vi "Example Callback - UVI Callback.vi"(4 "UVI":refnum<user-event>, 5 "Event Data":cluster{"sender":refnum<k24>, "uvi":i32}, 6 "Control Ref":refnum<k24>, 7 "Event Common Data":T1) -> ()   [LabVIEW 2010]
uses:
  C:/tf/play/labview/Tinkerforge.dll
  Tinkerforge.dll
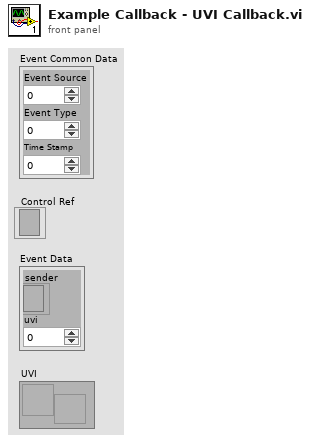
[diagram p1: front panel]
types:
  T1 = cluster{"Event Source":i32, "Event Type":u32, "Time Stamp":u32}
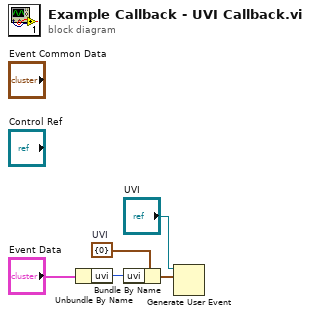
[diagram p0: block diagram]
diagram:
  w4 = cluster{"uvi":i32} {"uvi"=0}  # UVI
  n1 = Unbundle By Name("Event Data") -> ("uvi"=w3:i32)
  n2 = Bundle By Name(cluster=w4, "uvi"=w3) -> (w2:cluster{"uvi":i32})
  n3 = Generate User Event(user event="UVI", event data cluster=w2) -> ()  [unwired: 1 in, 2 out]
